vi "Archiver-Kill.vi"(8 "error in (no error)":errorcluster) -> (0 "error out":errorcluster)   [LabVIEW 2016]
uses:
  Archiver.Action.ctl
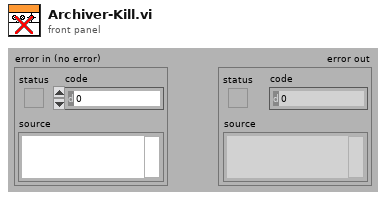
[diagram p1: front panel]
types:
  T1 = typedef "Archiver.Action.ctl" = enum32{"idle", "constructor", "destructor", "--- Archiver ---"}
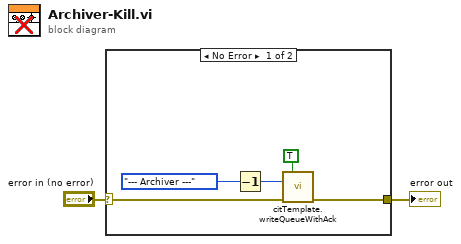
[diagram p0: block diagram]
diagram:
  n1 = case shown="No Error" "error in (no error)" {
    selector: "error in (no error)" -> [w7 w8]
    tunnel: [w6 w8] -> w1
    frame No Error {
      n2 = Decrement(x=Archiver.Action."--- Archiver ---" ("Action")) -> (x-1=w3:T1)
      n3 = call "citTemplate.writeQueueWithAck.vi"("High priority (F)"=TRUE, "event in"=w3, "error in (no error)"=w7) -> ("error out"=w6:errorcluster)  [unwired: 10 in, 2 out]
    }
    frame Error {
    }
  }
  "error out" <- w1
